vi "Read Default Name.vi"(8 "error in (no error)":errorcluster, 11 "Step UI in":refnum<class "Step UI.lvclass">) -> (0 "error out":errorcluster, 2 "Default Name":string, 3 "Step UI out":refnum<class "Step UI.lvclass">)   [LabVIEW 2015, in "Step UI.lvclass"]
uses:
  Step UI.lvclass
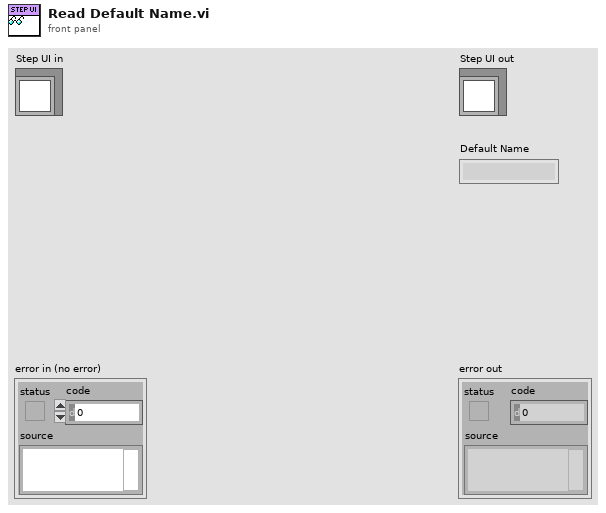
[diagram p1: front panel]
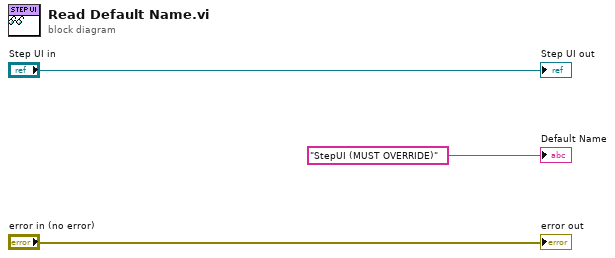
[diagram p0: block diagram]
diagram:
  "error out" <- "error in (no error)"
  "Step UI out" <- "Step UI in"
  "Default Name" <- "StepUI (MUST OVERRIDE)"
